vi "reprintsql.vi"(10 "pn":string, 11 "sn":string) -> (3 "exec sql":string)   [LabVIEW 2011]
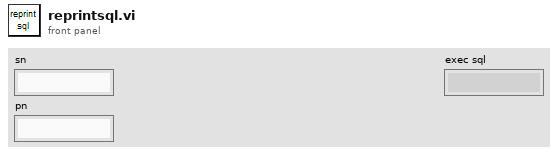
[diagram p1: front panel]
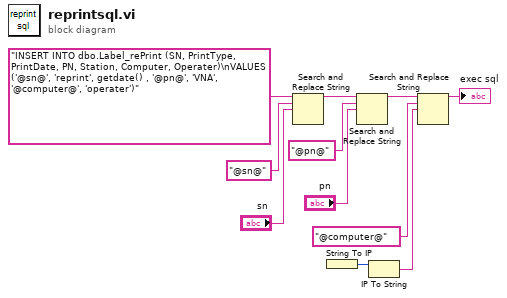
[diagram p0: block diagram]
diagram:
  n1 = Search and Replace String(input string="INSERT INTO dbo.Label_rePrint (SN, PrintType, PrintDate, PN, Station, Computer, Operater)\nVALUES ('@sn@', 'reprint', getdate() , '@pn@', 'VNA', '@computer@', 'operater')", search string="@sn@" ("搜索字符串"), replace string="sn") -> (result string=w8:string)  [unwired: 5 in, 3 out]
  n2 = String To IP() -> (0:w3:u32)  [unwired: 1 in]
  n3 = Search and Replace String(input string=w8, search string="@pn@" ("搜索字符串"), replace string="pn") -> (result string=w5:string)  [unwired: 5 in, 3 out]
  n4 = IP To String(2:w3) -> (0:w2:string)  [unwired: 1 in]
  n5 = Search and Replace String(input string=w5, search string="@computer@" ("搜索字符串"), replace string=w2) -> (result string=→"exec sql":string)  [unwired: 5 in, 3 out]
